vi "SwerveDrive.vi"(8 "error in (no error)":errorcluster) -> ()   [LabVIEW 2014]
uses:
  <vilib>/Rock Robotics/WPI/Joystick/WPI_JoystickGetSetRefNum.vi
panel:
  in  "Power Shaping Degree":dbl=2.0
  in  "Power Shaping Gain":dbl=50.0
  in  "Robot Width":dbl=36.25
  in  "Robot Length":dbl=24.5
  in  "EncoderTicksPerRev":dbl=1657.6
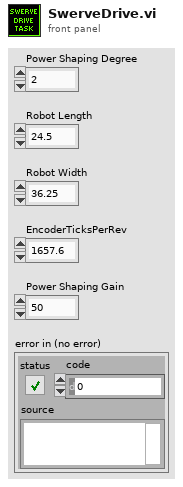
[diagram p1: front panel]
types:
  T1 = typedef "WPI_MotorControlDeviceRef.ctl" = cluster{"DeviceStatus":errorcluster, "Type":T2, "PWM":cluster{"Controller":T3, "PWM Channel":T4, "DeadBand":T5}, "CAN":cluster{"Device Number":u8, "Control Mode":T6, "Semaphore":T7, "Max Vout":dbl, "TalonSRX Control Mode":T8}, "Invert":bool, "TransformRef":T9, "InvTransformRef":T9}
  T2 = typedef "WPI_MotorControlType.ctl" = enum16{"PWM", "CAN", "CANTalonSRX"}
  T3 = typedef "FPGA_TypedefDigitalModule.ctl" = enum16{"Controller 1"}
  T4 = typedef "FPGA_DIOPWMChannel.ctl" = enum8{"PWM 0", "PWM 1", "PWM 2", "PWM 3", "PWM 4", "PWM 5", "PWM 6", "PWM 7", "PWM 8", "PWM 9", "PWM MXP 0", "PWM MXP 1", "PWM MXP 2", "PWM MXP 3", "PWM MXP 4", "PWM MXP 5", "PWM MXP 6", "PWM MXP 7", "PWM MXP 8", "PWM MXP 9", "Invalid"}
  T5 = typedef "WPI_PWMDeadband.ctl" = cluster{"Name":string, "maxPositivePwm":i32, "minPositivePwm":i32, "centerPwm":i32, "maxNegativePwm":i32, "minNegativePwm":i32, "angularRange":u16}
  T6 = typedef "WPI_CANJaguar_ControlMode.ctl" = enum8{"Percent VBus", "Current", "Speed", "Position", "Voltage"}
  T7 = typedef "Semaphore RefNum" = refnum<k1>
  T8 = typedef "WPI_CANTalonSRX_APIControlMode.ctl" = enum8{"Percent VBus", "Speed", "Position", "Slave", "Unchanged / Invalid"}
  T9 = typedef "WPI_PWMTransform_ConPane.ctl" = refnum<vi>
  T10 = typedef "WPI_JoystickDevRef.ctl" = cluster{"Device":T11}
  T11 = typedef "WPI_JoystickDeviceEnum.ctl" = enum16{"USB 0", "USB 1", "USB 2", "USB 3", "USB 4", "USB 5"}
  T12 = typedef "WPI_CANTalonSRX_GlobalStatus.ctl" = cluster{"Applied Throttle":dbl, "Module Enabled":bool, "CAN Error":errorcluster, "Closed Loop Error":dbl, "Forward Limit Switch Closed":bool, "Reverse Limit Switch Closed":bool, "Sensor Position":dbl, "Sensor Velocity":dbl, "Current":dbl, "Sticky Fault - Over Temp":bool, "Sticky Fault - Under Voltage":bool, "Sticky Fault - Forward Limit":bool, "Sticky Fault - Reverse Limit":bool, "Sticky Fault - Forward Soft Limit":bool, "Sticky Fault - Reverse Soft Limit":bool, "Brake is Enabled":bool, "Encoder Position":dbl, "Encoder Velocity":dbl, "Encoder Index Count":dbl, "Encoder A Pin State":bool, "Encoder B Pin State":bool, "Encoder Index Pin State":bool, "Analog In":dbl, "Analog In Velocity":dbl, "Temperature (C)":dbl, "Battery Voltage":dbl}
  T13 = typedef "WPI_I2CDevRef.ctl" = cluster{"DevStatus":errorcluster, "Controller":T3, "Device Address":u8, "Handle":i32, "I2C Bus":T14}
  T14 = typedef "i2c_bus.ctl" = enum16{"I2C On-Board", "I2C MXP", "Invalid"}
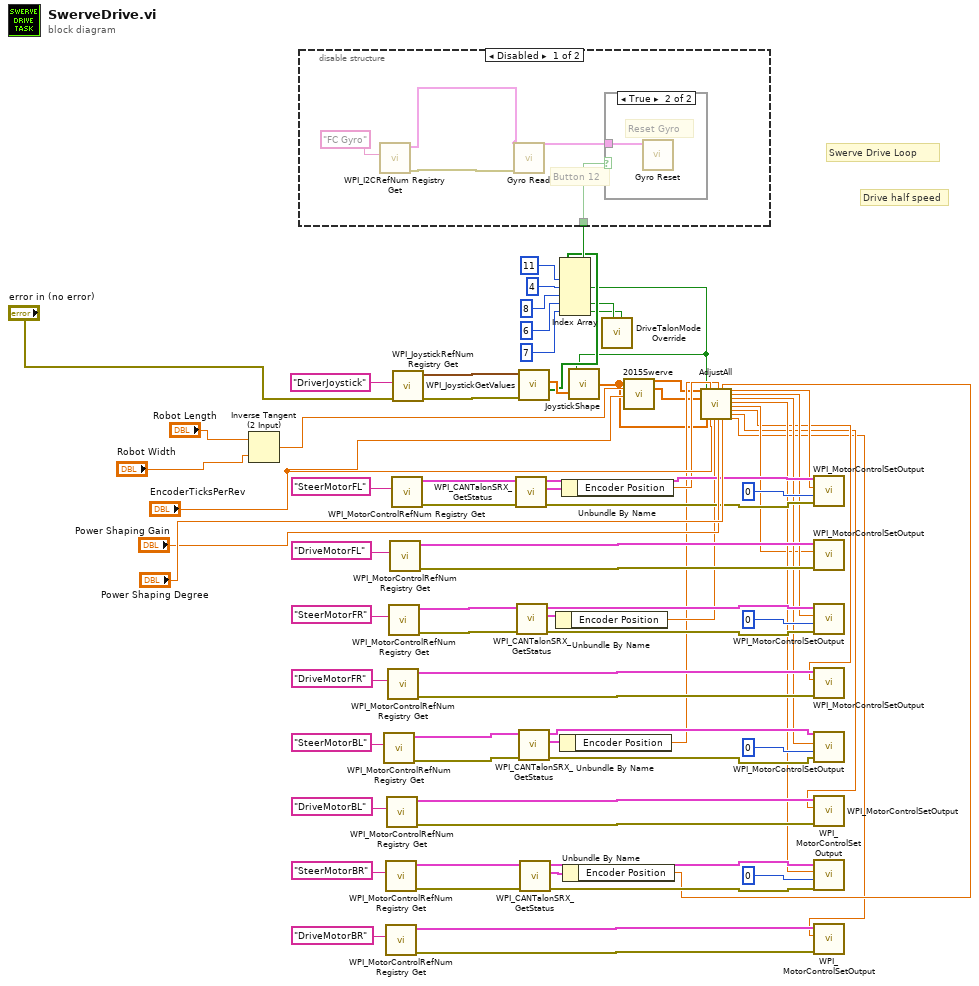
[diagram p0: block diagram]
diagram:
  # "Drive half speed"
  # "Swerve Drive Loop"
  n1 = Inverse Tangent (2 Input)(1:"Robot Width", 2:"Robot Length") -> (0:w71:dbl)
  n2 = call <vilib>:"WPI_MotorControlRefNum Registry Get.vi"("refnum name"="SteerMotorBL") -> ("error out"=w63:errorcluster, "MotorControlDevRef"=w62:T1)  [unwired: 9 in]
  n3 = call <vilib>:"WPI_MotorControlRefNum Registry Get.vi"("refnum name"="SteerMotorBR") -> ("error out"=w68:errorcluster, "MotorControlDevRef"=w67:T1)  [unwired: 9 in]
  n4 = call <vilib>:"WPI_MotorControlRefNum Registry Get.vi"("refnum name"="DriveMotorBR") -> ("error out"=w70:errorcluster, "MotorControlDevRef"=w69:T1)  [unwired: 9 in]
  n5 = call <vilib>:"WPI_MotorControlRefNum Registry Get.vi"("refnum name"="DriveMotorBL") -> ("error out"=w66:errorcluster, "MotorControlDevRef"=w65:T1)  [unwired: 9 in]
  n6 = call <vilib>:"WPI_MotorControlRefNum Registry Get.vi"("refnum name"="DriveMotorFR") -> ("error out"=w61:errorcluster, "MotorControlDevRef"=w60:T1)  [unwired: 9 in]
  n7 = call <vilib>:"WPI_MotorControlRefNum Registry Get.vi"("refnum name"="SteerMotorFR") -> ("error out"=w59:errorcluster, "MotorControlDevRef"=w58:T1)  [unwired: 9 in]
  n8 = call <vilib>:"WPI_MotorControlRefNum Registry Get.vi"("refnum name"="DriveMotorFL") -> ("error out"=w57:errorcluster, "MotorControlDevRef"=w56:T1)  [unwired: 9 in]
  n9 = call <vilib>:"WPI_MotorControlRefNum Registry Get.vi"("refnum name"="SteerMotorFL") -> ("error out"=w55:errorcluster, "MotorControlDevRef"=w54:T1)  [unwired: 9 in]
  n10 = call <vilib>:"WPI_JoystickRefNum Registry Get.vi"("error in (no error)"="error in (no error)", "refnum name"="DriverJoystick") -> ("error out"=w72:errorcluster, "JoystickDevRef"=w46:T10)  [unwired: 8 in]
  n11 = call <vilib>:"WPI_CANTalonSRX_GetStatus.vi"("error in (no error)"=w55, "CAN Talon SRX Ref"=w54) -> ("error out"=w38:errorcluster, "Talon SRX Status"=w37:T12, "CAN Talon SRX Ref Out"=w39:T1)  [unwired: 7 in]
  n12 = call <vilib>:"WPI_CANTalonSRX_GetStatus.vi"("error in (no error)"=w59, "CAN Talon SRX Ref"=w58) -> ("error out"=w35:errorcluster, "Talon SRX Status"=w34:T12, "CAN Talon SRX Ref Out"=w36:T1)  [unwired: 7 in]
  n13 = call <vilib>:"WPI_JoystickGetValues.vi"("error in (no error)"=w72, "JoystickDevRef"=w46) -> ("Buttons"=w18:bool[], "Axes"=w44:dbl[])  [unwired: 5 in, 3 out]
  n14 = call <vilib>:"WPI_CANTalonSRX_GetStatus.vi"("error in (no error)"=w63, "CAN Talon SRX Ref"=w62) -> ("error out"=w32:errorcluster, "Talon SRX Status"=w31:T12, "CAN Talon SRX Ref Out"=w33:T1)  [unwired: 7 in]
  n15 = call <vilib>:"WPI_CANTalonSRX_GetStatus.vi"("error in (no error)"=w68, "CAN Talon SRX Ref"=w67) -> ("error out"=w29:errorcluster, "Talon SRX Status"=w28:T12, "CAN Talon SRX Ref Out"=w30:T1)  [unwired: 7 in]
  n16 = Unbundle By Name(w34) -> ("Encoder Position"=w27:dbl)
  n17 = Index Array(array=w18, index #1=11 ("index"), index #2=4 ("index"), index #3=8 ("index"), index #4=6 ("index"), index #5=7 ("index")) -> (element #1=w19:bool, element #2=w1:bool, element #4=w6:bool, element #5=w4:bool)  [unwired: 1 out]
  n18 = disable-structure shown="Disabled" {
    disable-tunnel: w19 -> [w77 _]
    frame Disabled {
      # "Button 12"
      n19 = call <vilib>:"WPI_I2CRefNum Registry Get.vi"("refnum name"="FC Gyro") -> ("error out"=w80:errorcluster, "I2CDevRef"=w79:T13)  [unwired: 9 in]
      n20 = call "Gyro Read.vi"("error in (no error)"=w80, "I2CDevRef In"=w79) -> ()  [unwired: 7 in, 3 out]
      n21 = case shown="True" w77 {
        tunnel: w79 -> [_ w81]
        frame False {
        }
        frame True {
          # "Reset Gyro"
          n22 = call "Gyro Reset.vi"("I2CDevRef"=w81) -> ()  [unwired: 10 in, 1 out]
        }
      }
    }
    frame Enabled {
    }
  }
  n23 = Unbundle By Name(w31) -> ("Encoder Position"=w25:dbl)
  n24 = Unbundle By Name(w37) -> ("Encoder Position"=w26:dbl)
  n25 = Unbundle By Name(w28) -> ("Encoder Position"=w24:dbl)
  n26 = call "JoystickShape.vi"("JoystickValues"=w44, "SlowSpeed"=w1) -> ("JoystickOut"=w13:dbl[])
  n27 = call "DriveTalonModeOverride.vi"("Coast"=w4, "Brake"=w6) -> ()  [unwired: 10 in]
  n28 = call "2015Swerve.vi"("Axes"=w13, "Robot Dimension Calc"=w71, "EncoderTicksPerRev"="EncoderTicksPerRev") -> ("SteeringArray"=w15:dbl[], "PowerArray"=w14:dbl[])  [unwired: 23 in]
  n29 = call "AdjustAll.vi"("SteeringAngleArray"=w15, "PowerArray"=w14, "Third Speed"=w1, "JoystickValues"=w13, "FL Enc"=w26, "EncoderTicksPerRev"="EncoderTicksPerRev", "FR Enc"=w27, "BL Enc"=w25, "Gain"="Power Shaping Gain", "BR Enc"=w24, "Shaping Degree"="Power Shaping Degree") -> ("FL Set Out"=w23:dbl, "FR Set Out"=w22:dbl, "BL Set Out"=w21:dbl, "BR Set Out"=w20:dbl, "FL Power"=w12:dbl, "FR Power"=w11:dbl, "BL Power"=w10:dbl, "BR Power"=w9:dbl)  [unwired: 9 in]
  n30 = call <vilib>:"WPI_MotorControlSetOutput.vi"("error in (no error)"=w38, "Sync Group / Parameter Slot"=u8 0, "Output"=w23, "MotorControlDevRef"=w39) -> ()  [unwired: 5 in, 3 out]
  n31 = call <vilib>:"WPI_MotorControlSetOutput.vi"("error in (no error)"=w57, "Output"=w12, "MotorControlDevRef"=w56) -> ()  [unwired: 6 in, 3 out]
  n32 = call <vilib>:"WPI_MotorControlSetOutput.vi"("error in (no error)"=w35, "Sync Group / Parameter Slot"=u8 0, "Output"=w22, "MotorControlDevRef"=w36) -> ()  [unwired: 5 in, 3 out]
  n33 = call <vilib>:"WPI_MotorControlSetOutput.vi"("error in (no error)"=w61, "Output"=w11, "MotorControlDevRef"=w60) -> ()  [unwired: 6 in, 3 out]
  n34 = call <vilib>:"WPI_MotorControlSetOutput.vi"("error in (no error)"=w32, "Sync Group / Parameter Slot"=u8 0, "Output"=w21, "MotorControlDevRef"=w33) -> ()  [unwired: 5 in, 3 out]
  n35 = call <vilib>:"WPI_MotorControlSetOutput.vi"("error in (no error)"=w66, "Output"=w10, "MotorControlDevRef"=w65) -> ()  [unwired: 6 in, 3 out]
  n36 = call <vilib>:"WPI_MotorControlSetOutput.vi"("error in (no error)"=w29, "Sync Group / Parameter Slot"=u8 0, "Output"=w20, "MotorControlDevRef"=w30) -> ()  [unwired: 5 in, 3 out]
  n37 = call <vilib>:"WPI_MotorControlSetOutput.vi"("error in (no error)"=w70, "Output"=w9, "MotorControlDevRef"=w69) -> ()  [unwired: 6 in, 3 out]
